vi "FYP_VI_MIDI_InstrumentSelect.vi"(5 "MIDI Channel":u32 max=15, 6 "Instrument":u32 max=127, 7 "midiOut handle":i32) -> (0 "midiOutShortMsg Error Code":i32, 3 "midiOut handle":i32)   [LabVIEW 2013]
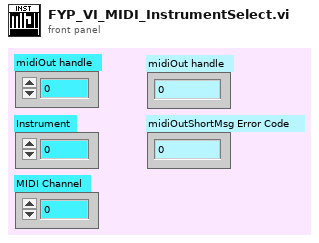
[diagram p1: front panel]
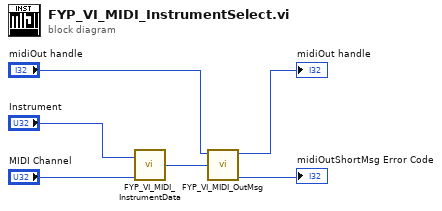
[diagram p0: block diagram]
diagram:
  n1 = call "FYP_VI_MIDI_InstrumentData.vi"("MIDI Channel"="MIDI Channel", "Instrument"="Instrument") -> ("MIDI Instrument data"=w4:u32)
  n2 = call "FYP_VI_MIDI_OutMsg.vi"("dwMsg dataIn"=w4, "midiOut hmo"="midiOut handle") -> ("midiOutShortMsg Error Code"=→"midiOutShortMsg Error Code":i32, "midiOut handle"=→"midiOut handle":i32)  [unwired: 4 in]
